vi "更改输入顺序4字节.vi"(10 "输入数据":u16[](array[numeric])) -> (2 "更改顺序后数据":u16[](array[numeric]))   [LabVIEW 2010]
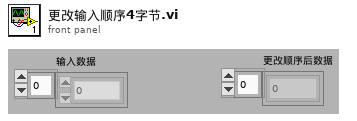
[diagram p1: front panel]
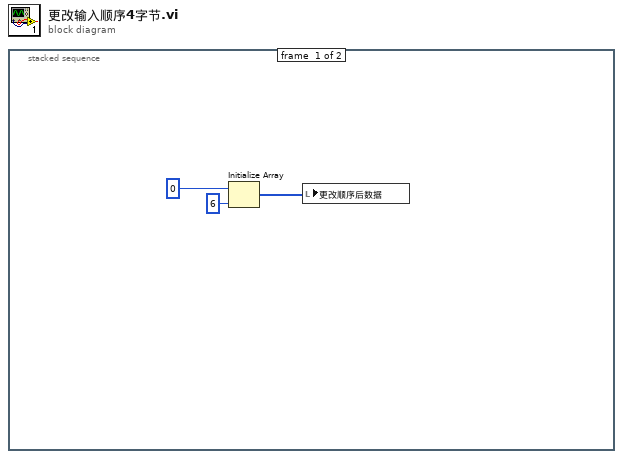
[diagram p0: block diagram]
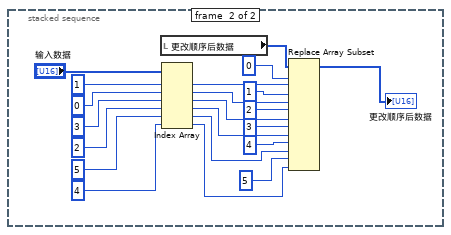
[diagram p2: hidden frame]
diagram:
  n1 = stacked-sequence {
    frame #0 {
      n2 = Initialize Array(u16 0, 6 ("维数大小")) -> (w1:u16[])
      n3 = local write "更改顺序后数据"(w1) -> ()
    }
    frame #1 {
      n4 = local read "更改顺序后数据"() -> (w19:u16[])
      n5 = Index Array(array="输入数据", index #1=1 ("索引"), index #2=0 ("索引"), index #3=3 ("索引"), index #4=2 ("索引"), index #5=5 ("索引"), index #6=4 ("索引")) -> (element #1=w17:u16, element #2=w15:u16, element #3=w14:u16, element #4=w11:u16, element #5=w7:u16, element #6=w6:u16)
      n6 = Replace Array Subset(array=w19, new element #1=w17, index #1=0 ("索引"), new element #2=w15, index #2=1 ("索引"), new element #3=w14, index #3=2 ("索引"), new element #4=w11, index #4=3 ("索引"), new element #5=w7, index #5=4 ("索引"), new element #6=w6, index #6=5 ("索引")) -> (→"更改顺序后数据":u16[])
    }
  }
